vi "checkMotorOverheat.vi"(8 "error in (no error)":errorcluster, 11 "MotorTemperatureSensor in":refnum<class "MotorTemperatureSensor.lvclass">) -> (0 "error out":errorcluster, 2 "motorOverheatActiveIsTrue":bool, 3 "MotorTemperatureSensor out":refnum<class "MotorTemperatureSensor.lvclass">)   [LabVIEW 2013, in "MotorTemperatureSensor.lvclass"]
uses:
  MotorTemperatureSensor.lvclass
  <userlib>/Common/Devices/TemperatureSensor/TemperatureSensor/TemperatureSensor.lvclass/TemperatureSensor.ctl
  MotorTemperatureSensor.lvclass/MotorTemperatureSensor.ctl
  <userlib>/Common/Devices/TemperatureSensor/TemperatureSensor/TemperatureSensor.lvclass
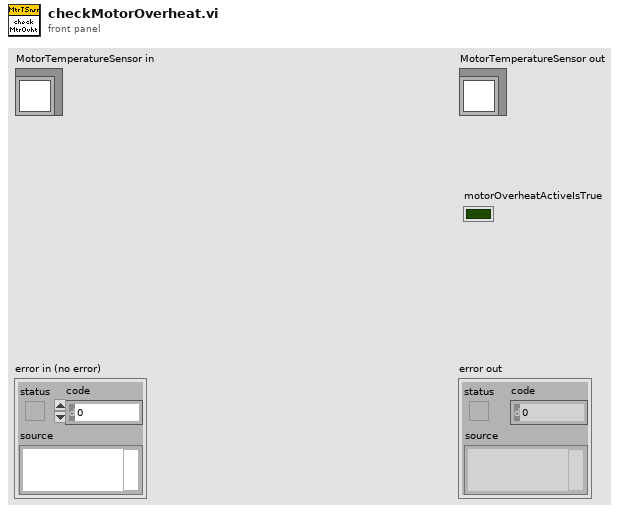
[diagram p1: front panel]
types:
  T1 = typedef "MotorOverheatTemperature.ctl" = dbl[unit]
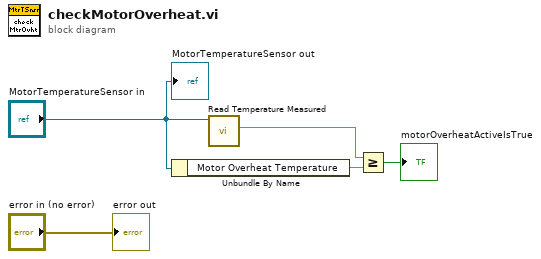
[diagram p0: block diagram]
diagram:
  n1 = Unbundle By Name("MotorTemperatureSensor in") -> ("Motor Overheat Temperature"=w2:T1)
  n2 = call <userlib>:"Read Temperature Measured.vi"("TemperatureSensor in"="MotorTemperatureSensor in") -> ("Temperature Measured"=w3:dbl[unit])  [unwired: 9 in, 1 out]
  n3 = Greater Or Equal?(x=w3, y=w2) -> (x >= y?=→"motorOverheatActiveIsTrue":bool)
  "error out" <- "error in (no error)"
  "MotorTemperatureSensor out" <- "MotorTemperatureSensor in"
